vi "Turn To X.vi"(0 "FPGA VI Reference in":refnum<k20>, 1 "STOP?":bool, 2 "error in":errorcluster, 3 "Start":u16, 5 "Dest":u16) -> (6 "FPGA VI Reference Out":refnum<k20>, 7 "x-y":i16, 8 "error out":errorcluster)   [LabVIEW 2014]
uses:
  <vilib>/Utility/error.llb/Error Cluster From Error Code.vi
  <vilib>/rvi/errors/niLvFpgaAdjustHostInterfaceError.vi
  <vilib>/rvi/interface/nirviReadWriteControl/nirviReadWriteControl.xnode
  NiFpgaLv.dll
  <vilib>/rvi/interface/Simulation/niFpgaSimulationCallBeginRW.vi
panel:
  out "Move Stop":bool
  out "16bit integer":i16
  in  "Friction":dbl=1.0
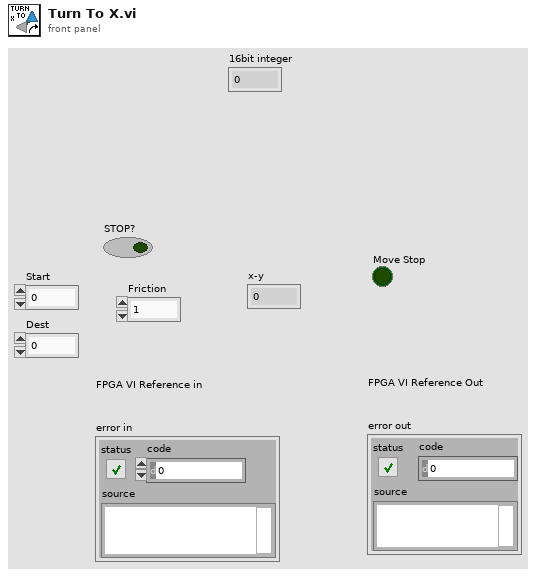
[diagram p1: front panel]
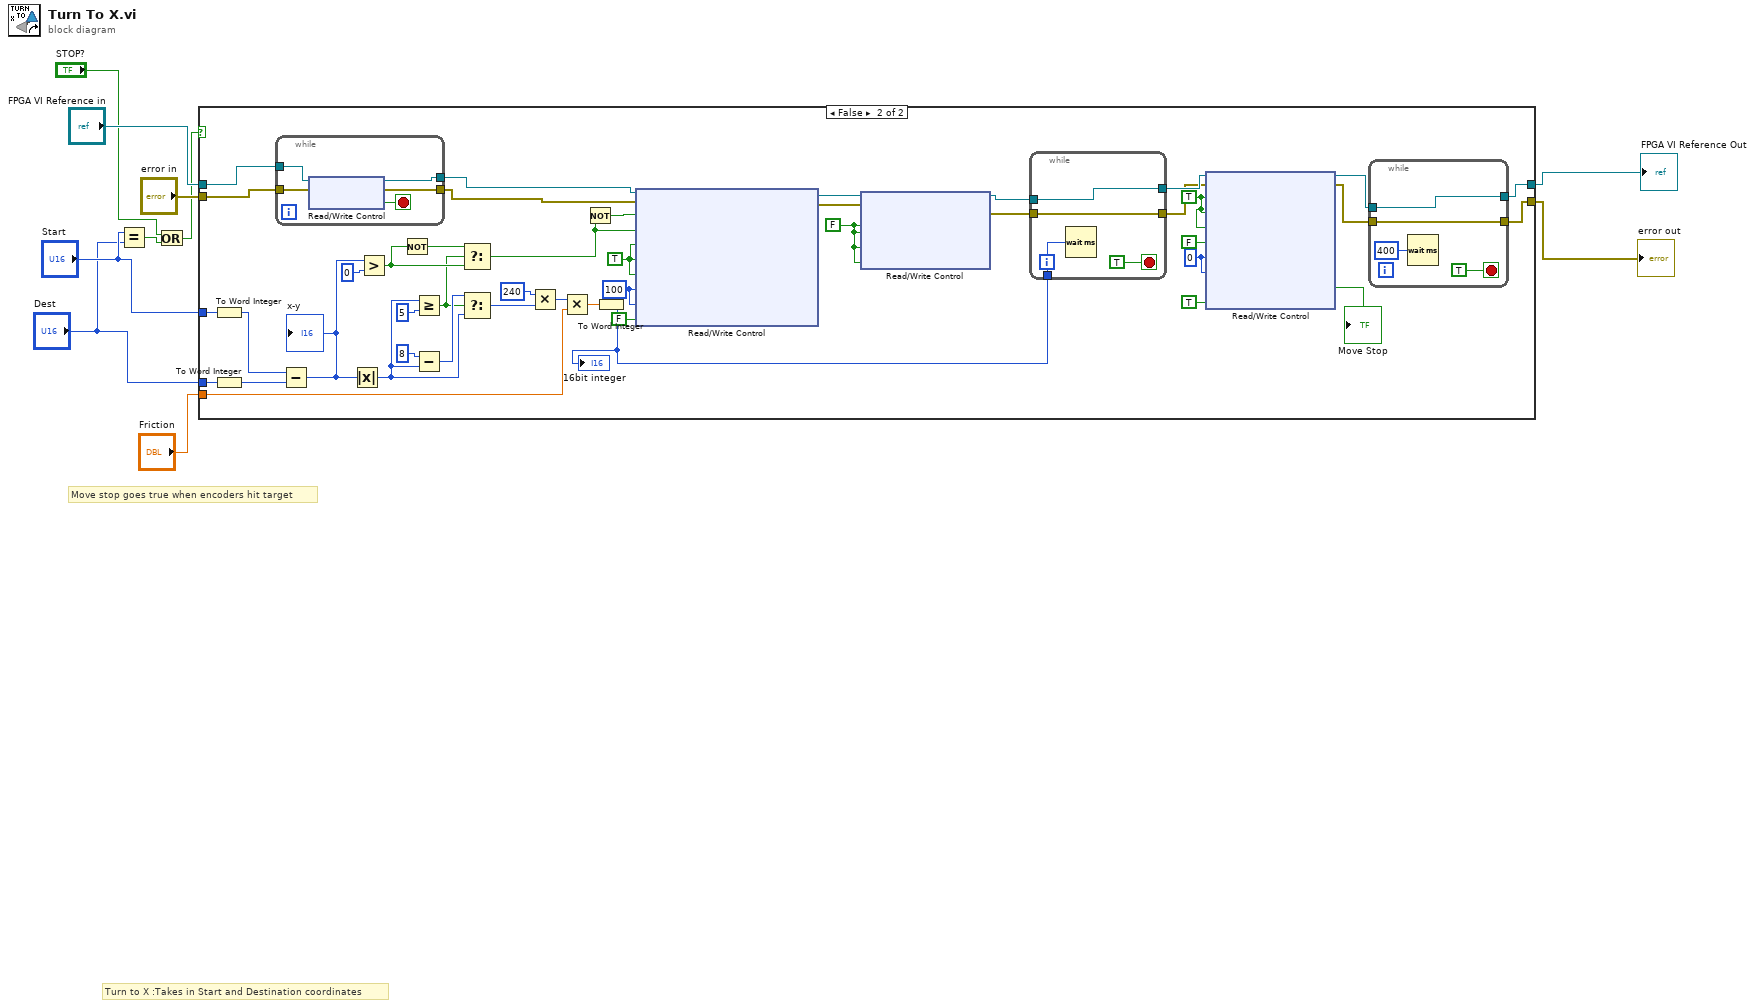
[diagram p0: block diagram]
diagram:
  # "Move stop goes true when encoders hit target"
  # "Turn to X :Takes in Start and Destination coordinates"
  n1 = Equal?(x="Start", y="Dest") -> (x = y?=w3:bool)
  n2 = Or(x="STOP?", y=w3) -> (x .or. y?=w1:bool)
  n3 = case shown="False" w1 {
    tunnel: "Start" -> [_ w55]
    tunnel: "Dest" -> [_ w52]
    tunnel: "error in" -> [w11 w24]
    tunnel: "FPGA VI Reference in" -> [w12 w25]
    tunnel: [w12 w21] -> w8
    tunnel: [w11 w20] -> w7
    tunnel: "Friction" -> [_ w56]
    frame True {
    }
    frame False {
      w19 = u32 100 ("Left motor pulse width (uSec)")
      w29 = i16 0 ("Left Count Length")
      w28 = TRUE ("Stop Left")
      w30 = FALSE ("Stop Left")
      w31 = TRUE ("Right Motor")
      n4 = To Word Integer(number=w55) -> (16bit integer=w54:i16)
      n5 = To Word Integer(number=w52) -> (16bit integer=w53:i16)
      n6 = while {
        tunnel: [w64] -> w26
        tunnel: [w63] -> w27
        tunnel: w25 -> [w62]
        tunnel: w24 -> [w61]
        stop <- w65 stop-if-true
        n7 = xnode "Read/Write Control"("FPGA VI Reference In"=w62, "error in"=w61) -> ("FPGA VI Reference Out"=w63:refnum<k20>, "error out"=w64:errorcluster, "Move Stop"=w65:bool)
      }
      n8 = Subtract(x=w54, y=w53) -> (x-y=w49:i16)
      "x-y" <- w49
      n9 = Absolute Value(x=w49) -> (abs(x)=w37:i16)
      n10 = Greater?(x=w49, y=i16 0) -> (0:w40:bool)
      n11 = Not(x=w40) -> (.not. x?=w41:bool)
      n12 = Greater Or Equal?(x=w37, y=i16 5 ("x")) -> (x >= y?=w39:bool)
      n13 = Subtract(x=i16 8, y=w37) -> (x-y=w44:i16)
      n14 = Select(t=w41, s=w39, f=w40) -> (s? t:f=w17:bool)
      n15 = Select(t=w44, s=w39, f=w37) -> (s? t:f=w42:i16)
      n16 = Multiply(x=240 ("y"), y=w42) -> (x*y=w48:i32)
      n17 = Multiply(x=w48, y=w56) -> (x*y=w50:dbl)
      n18 = Not(x=w17) -> (.not. x?=w18:bool)
      n19 = To Word Integer(number=w50) -> (16bit integer=w34:i16)
      "16bit integer" <- w34
      n20 = xnode "Read/Write Control"("FPGA VI Reference In"=w27, "error in"=w26, "Left Motor"=w18, "Right Motor"=w17, "Stop Left"=w31, "Stop Right"=w31, "reset wheel count (T)"=w31, "Left motor pulse width (uSec)"=w19, "Right motor pulse width (uSec)"=w19, "Smart Stop"=FALSE) -> ("FPGA VI Reference Out"=w47:refnum<k20>, "error out"=w46:errorcluster)
      n21 = xnode "Read/Write Control"("FPGA VI Reference In"=w47, "error in"=w46, "Stop Left"=w30, "Stop Right"=w30, "Stop motors"=w30, "reset wheel count (T)"=w30) -> ("FPGA VI Reference Out"=w36:refnum<k20>, "error out"=w35:errorcluster)
      n22 = while {
        tunnel: [w69] -> w33
        tunnel: w36 -> [w69]
        tunnel: [w68] -> w32
        tunnel: w35 -> [w68]
        tunnel: w34 -> [w66]
        stop <- TRUE stop-if-true
        n23 = Wait (ms)(milliseconds to wait=w66) -> ()  [unwired: 1 out]
      }
      n24 = xnode "Read/Write Control"("FPGA VI Reference In"=w33, "error in"=w32, "Stop Left"=w28, "Stop Right"=w28, "Stop motors"=w28, "reset wheel count (T)"=FALSE, "Left Count Length"=w29, "Right Count Length"=w29, "Smart Stop"=TRUE) -> ("FPGA VI Reference Out"=w23:refnum<k20>, "error out"=w22:errorcluster, "Move Stop"=→"Move Stop":bool)
      n25 = while {
        tunnel: [w60] -> w21
        tunnel: w23 -> [w60]
        tunnel: [w59] -> w20
        tunnel: w22 -> [w59]
        stop <- TRUE stop-if-true
        n26 = Wait (ms)(milliseconds to wait=u32 400) -> ()  [unwired: 1 out]
      }
    }
  }
  "FPGA VI Reference Out" <- w8
  "error out" <- w7
